vi "ReadRecorderStatus.vi"(4 "error in (no error)":errorcluster, 7 "axis in":cluster{"keyHandle":u32, "nodeId":u16}={"keyHandle"=0, "nodeId"=1}) -> (0 "error out":errorcluster, 1 "isRunning":i32, 2 "isTriggered":i32, 3 "axis out":cluster{"keyHandle":u32, "nodeId":u16}={"keyHandle"=0, "nodeId"=1})   [LabVIEW 2018]
doc: "<B>ReadRecorderStatus</B> reads the trigger state and if the data recorder is running."
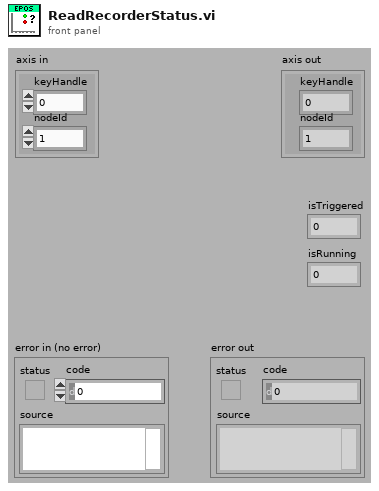
[diagram p1: front panel]
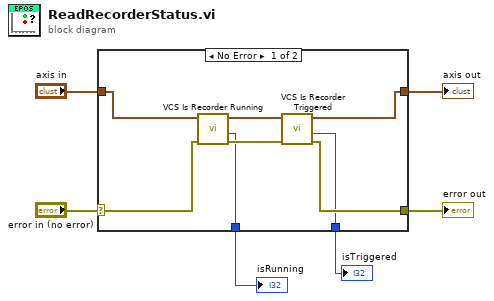
[diagram p0: block diagram]
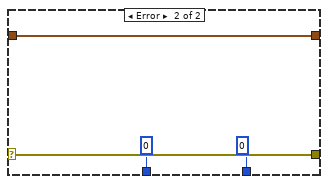
[diagram p2: hidden frame]
diagram:
  n1 = case shown="No Error" "error in (no error)" {
    selector: "error in (no error)" -> [w11 w18]
    tunnel: [w13 w18] -> w5
    tunnel: [w14 w17] -> w4
    tunnel: "axis in" -> [w10 w17]
    tunnel: [w8 0 ("isTriggered")] -> w2
    tunnel: [w7 0 ("isRunning")] -> w1
    frame No Error {
      n2 = call "VCS Is Recorder Running.vi"("error in (no error)"=w11, "axis in"=w10) -> ("error out"=w12:errorcluster, "isRunning"=w7:i32, "axis out"=w9:cluster{"keyHandle":u32, "nodeId":u16})  [unwired: 7 in]
      n3 = call "VCS Is Recorder Triggered.vi"("error in (no error)"=w12, "axis in"=w9) -> ("error out"=w13:errorcluster, "isTriggered"=w8:i32, "axis out"=w14:cluster{"keyHandle":u32, "nodeId":u16})  [unwired: 7 in]
    }
    frame Error {
    }
  }
  "error out" <- w5
  "axis out" <- w4
  "isRunning" <- w1
  "isTriggered" <- w2
